vi "PH_Beckhoff_Watchdog.ProcEvents.vi"(0 "i ref in":refnum<vi>, 5 "error in (no error)":errorcluster) -> (14 "i ref out":refnum<vi>, 19 "error out":errorcluster)   [LabVIEW 2014, in "PH_Beckhoff_Watchdog.lvlib"]
doc: "This method is used to define the events the object will listen to. Add your own events here."
uses:
  PH_Beckhoff_Watchdog.lvlib
  PH_Basics/PH_Common/DIM/PH_DIM.Event Declarer.ctl
  CS_Core/BaseProcess/BaseProcess.lvlib
  PH_Basics/PH_Common/PH_Common.lvlib
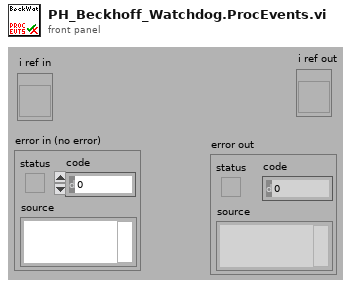
[diagram p1: front panel]
types:
  T1 = typedef "PH_Common.lvlib/PH_DIM.Event Declarer.ctl" = cluster{"Service Name":string, "Selector":string}
  T2 = typedef "PH_Beckhoff_Watchdog.lvlib/PH_Beckhoff_Watchdog.i attribute.ctl" = cluster{"Info":cluster{"GUI Ref":refnum<vi>, "Status":T3}[]}
  T3 = typedef "PH_StatusHandler.lvlib/PH_StatusHandler.Status.ctl" = i16
  T4 = typedef "BaseProcess.lvlib/BaseProcess.event definition.ctl" = cluster{"CAEEvtDef":T5, "Data Descriptor":T6}
  T5 = typedef "CAEObj.lvlib/CAEObj.event definition.ctl" = cluster{"URL":string, "enable":bool, "ignoreResID":bool}
  T6 = typedef "BaseProcess.lvlib/BaseProcess.descriptor string definition.ctl" = string
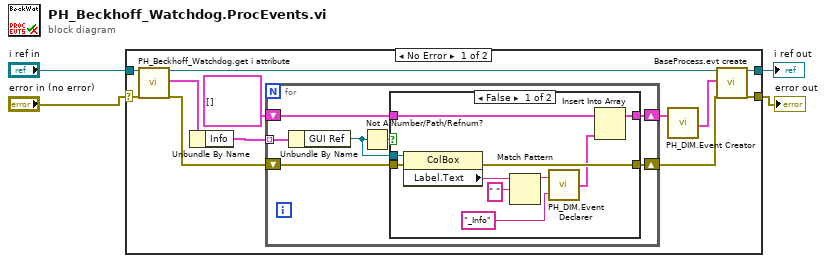
[diagram p0: block diagram]
diagram:
  n1 = case shown="No Error" "error in (no error)" {
    selector: "error in (no error)" -> [w11 w37]
    tunnel: "i ref in" -> [w13 w36]
    tunnel: [w16 w36] -> w3
    tunnel: [w15 w37] -> w2
    frame No Error {
      n2 = call "PH_Beckhoff_Watchdog.get i attribute.vi"("i ref in"=w13, "error in (no error)"=w11) -> ("i ref out"=w12:refnum<vi>, "i attribute"=w14:T2, "error out"=w7:errorcluster)  [unwired: 15 in]
      n3 = Unbundle By Name(w14) -> ("Info"=w5:cluster{"GUI Ref":refnum<vi>, "Status":T3}[])
      n4 = for {
        tunnel: w5 -> [w18] mode=indexing
        shift-right: [w22] -> w10
        shift-left: w7 -> [w23]
        shift-right: [w19] -> w6
        shift-left: T1[] [] -> [w20]
        n5 = Unbundle By Name(w18) -> ("GUI Ref"=w17:refnum<vi>)
        n6 = Not A Number/Path/Refnum?(number/path/refnum=w17) -> (NaN/Path/Refnum?=w21:bool)
        n7 = case shown="False" w21 {
          tunnel: [w33 w35] -> w22
          tunnel: w23 -> [w32 w35]
          tunnel: w17 -> [w31 _]
          tunnel: w20 -> [w30 w34]
          tunnel: [w29 w34] -> w19
          frame False {
            n8 = property class="ColBox"(reference=w31, error in=w32) -> (error out=w33:errorcluster, "Label.Text"=w27:string)  [unwired: 1 out]
            n9 = Match Pattern(string=w27, regular expression=" ") -> (before substring=w26:string)  [unwired: 1 in, 3 out]
            n10 = call "PH_DIM.Event Declarer.vi"("Selector"="_Info", "Service Name"=w26) -> ("declared DIM Event"=w25:T1)
            n11 = Insert Into Array(array=w30, new element=w25) -> (w29:T1[])  [unwired: 1 in]
          }
          frame True {
          }
        }
      }
      n12 = call "PH_DIM.Event Creator.vi"("Trendmessage Services"=w6) -> ("DIM Service Events"=w8:T4[])  [unwired: 18 in]
      n13 = call "BaseProcess.evt create.vi"("i ref in"=w12, "newEvents"=w8, "error in (no error)"=w10) -> ("i ref out"=w16:refnum<vi>, "error out"=w15:errorcluster)  [unwired: 13 in, 2 out]
    }
    frame Error {
    }
  }
  "i ref out" <- w3
  "error out" <- w2
